vi "Latihan soal UTS 2020.vi"() -> ()   [LabVIEW 2020]
panel:
  out "Warning Counter":i32
  in  "Operator":string
  out "WARNING":bool
  out "Waveform Chart":T1(graph)
  out "START/STOP":bool
  in  "STOP":bool
  in  "START/STOP":bool
  in  "C   or   F":bool
  in  "HIGH Limit":dbl(slide) scale=0.0..100.0
  in  "LOW Limit":dbl(slide) scale=0.0..100.0
  in  "Filename":path
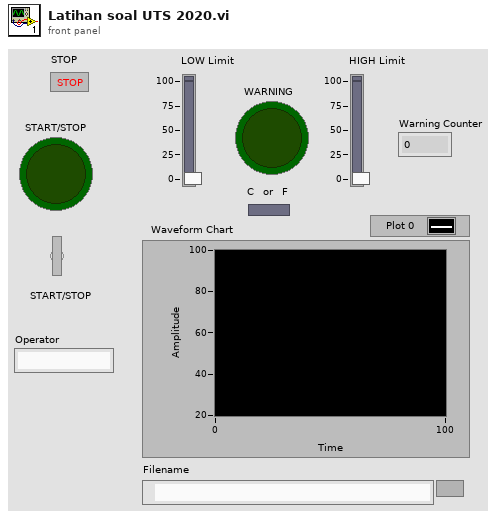
[diagram p1: front panel]
types:
  T1 = cluster{"Temperature (deg F)":dbl, "LOW Limit":dbl, "HIGH Limit":dbl}
  T2 = enum16{"open", "replace", "create", "open or create", "replace or create", "replace or create with confirmation"}
  T3 = cluster{"Y":dbl, "LOW Limit":dbl, "HIGH Limit":dbl}
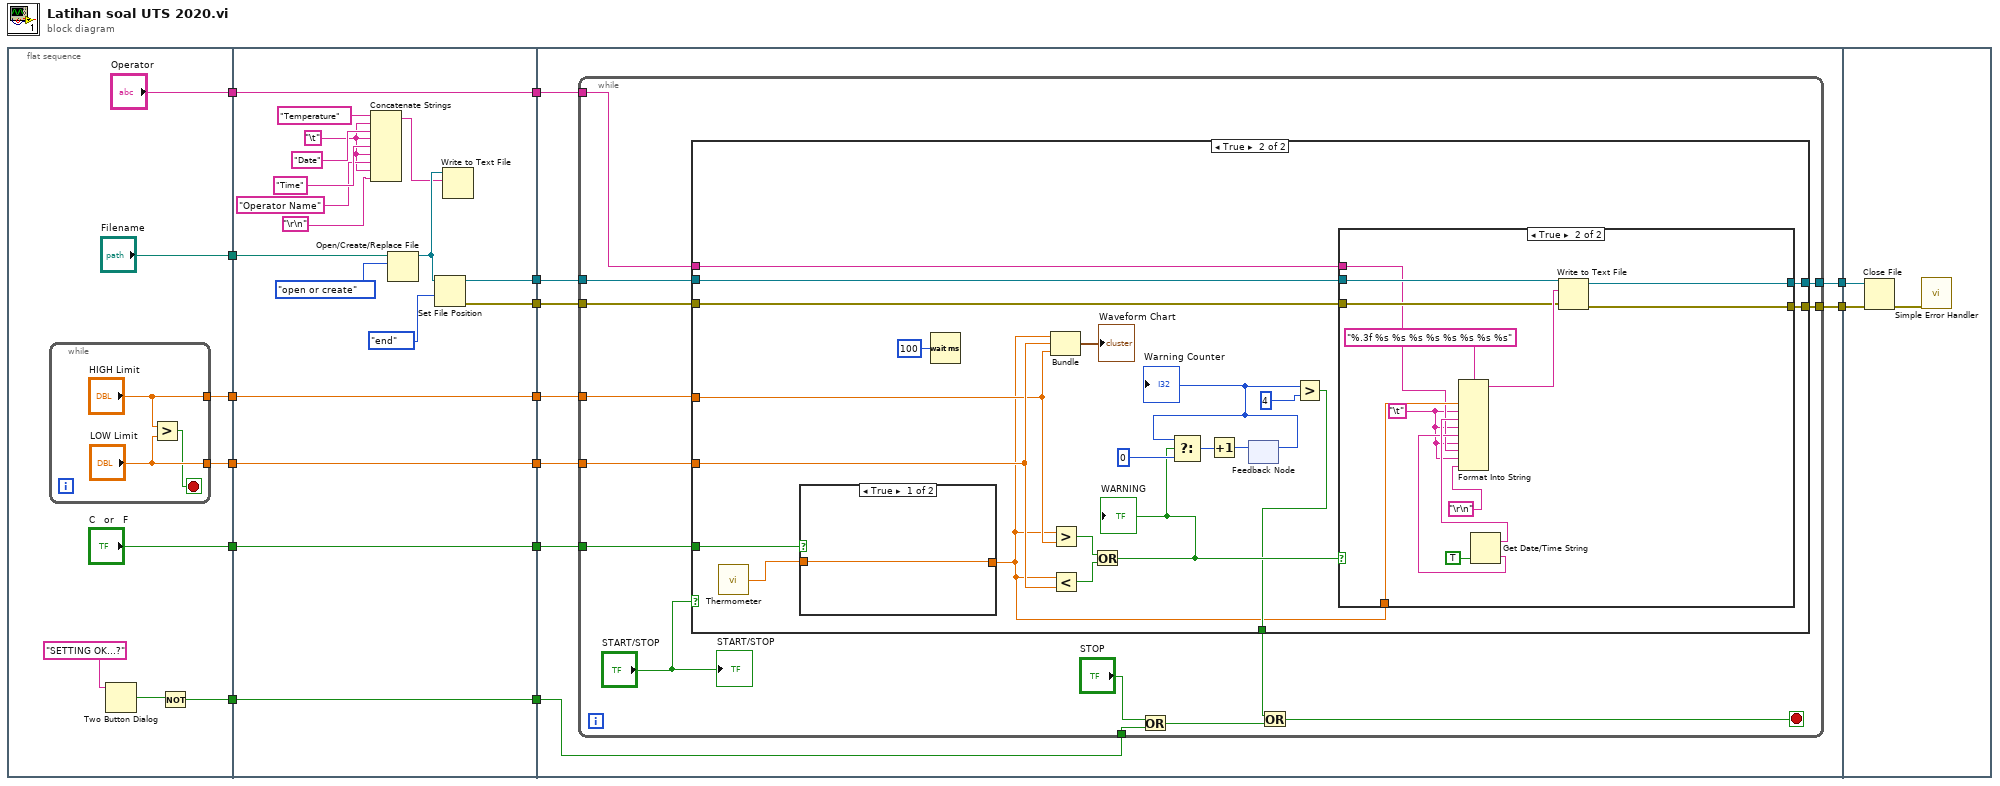
[diagram p0: block diagram]
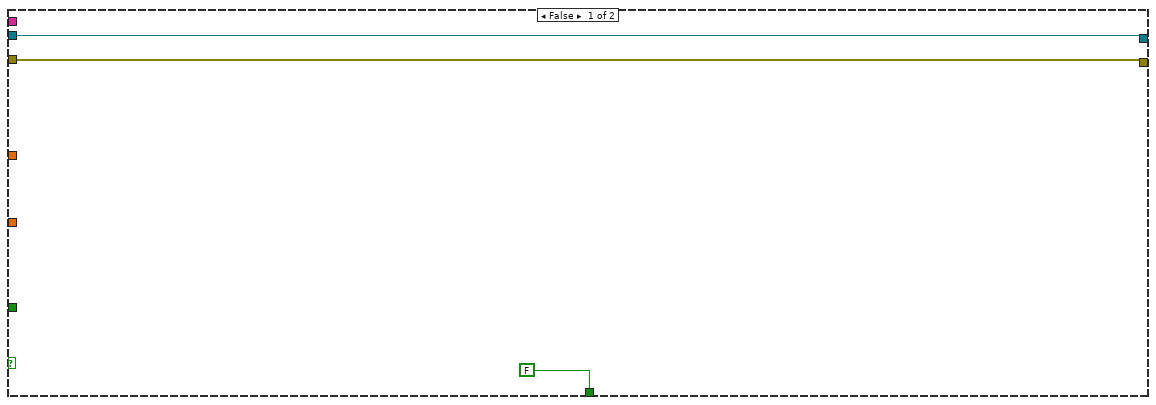
[diagram p2: hidden frame]
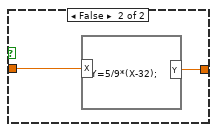
[diagram p4: hidden frame]
diagram:
  n1 = flat-sequence {
    tunnel: ["Filename"] -> w15
    tunnel: ["C   or   F"] -> w13
    tunnel: [w16] -> w11
    tunnel: [w19] -> w9
    tunnel: [w17] -> w3
    tunnel: ["Operator"] -> w1
    tunnel: w15 -> [w44]
    tunnel: [w42] -> w14
    tunnel: w13 -> [w42]
    tunnel: [w28] -> w12
    tunnel: w11 -> [w28]
    tunnel: [w41] -> w10
    tunnel: w9 -> [w41]
    tunnel: [w40] -> w8
    tunnel: [w39] -> w7
    tunnel: [w29] -> w4
    tunnel: w3 -> [w29]
    tunnel: [w36] -> w2
    tunnel: w1 -> [w36]
    tunnel: w14 -> [w53]
    tunnel: w12 -> [w52]
    tunnel: w10 -> [w51]
    tunnel: w8 -> [w50]
    tunnel: w7 -> [w49]
    tunnel: [w48] -> w6
    tunnel: [w47] -> w5
    tunnel: w4 -> [w46]
    tunnel: w2 -> [w45]
    tunnel: w6 -> [w112]
    tunnel: w5 -> [w111]
    frame #0 {
      n2 = while {
        tunnel: ["HIGH Limit"] -> w17
        tunnel: ["LOW Limit"] -> w16
        stop <- w24 stop-if-true
        n3 = Greater?(x="HIGH Limit", y="LOW Limit") -> (0:w24:bool)
      }
      n4 = Two Button Dialog(message="SETTING OK...?") -> (T button?=w20:bool)  [unwired: 2 in]
      n5 = Not(x=w20) -> (.not. x?=w19:bool)
    }
    frame #1 {
      w27 = "\t"
      n6 = Concatenate Strings("Temperature" ("string"), w27, "Date" ("string"), w27, "Time" ("string"), w27, "Operator Name" ("string"), w27, "\r\n") -> (w35:string)
      n7 = Open/Create/Replace File(file path (use dialog)=w44, operation (0:open)=T2."open or create") -> (refnum out=w38:refnum<file>)  [unwired: 4 in, 2 out]
      n8 = Set File Position(refnum=w38, from (0:start)=enum16{"start", "end", "current"}."end") -> (refnum out=w40:refnum<file>, error out=w39:errorcluster)  [unwired: 2 in]
      n9 = Write to Text File(file (use dialog)=w38, text=w35) -> ()  [unwired: 2 in, 3 out]
    }
    frame #2 {
      n10 = while {
        tunnel: w53 -> [w67]
        tunnel: w52 -> [w66]
        tunnel: w51 -> [w64]
        tunnel: w50 -> [w63]
        tunnel: w49 -> [w62]
        tunnel: [w61] -> w48
        tunnel: [w60] -> w47
        tunnel: w46 -> [w59]
        tunnel: w45 -> [w58]
        stop <- w56 stop-if-true
        n11 = case shown="True" "START/STOP" {
          tunnel: w67 -> [_ w91]
          tunnel: w59 -> [_ w76]
          tunnel: w66 -> [_ w81]
          tunnel: w63 -> [w70 w86]
          tunnel: w62 -> [w69 w85]
          tunnel: [w70 w84] -> w61
          tunnel: [w69 w83] -> w60
          tunnel: w58 -> [_ w82]
          tunnel: [FALSE w74] -> w55
          frame False {
          }
          frame True {
            n12 = call "Thermometer.vi"() -> ("Temperature (deg F)"=w71:dbl)  [unwired: 1 in]
            n13 = case shown="True" w91 {
              tunnel: w71 -> [w107 w109]
              tunnel: [w107 w108] -> w72
              frame True {
              }
              frame False {
                n14 = formula code="Y=5/9*(X-32);"("X"=w109) -> ("Y"=w108:dbl)
              }
            }
            n15 = Wait (ms)(milliseconds to wait=u32 100) -> ()  [unwired: 1 out]
            n16 = Bundle("Y"=w72, "LOW Limit"=w81, "HIGH Limit"=w76) -> (→"Waveform Chart":T3)  [unwired: 1 in]
            n17 = Greater?(x=w72, y=w76) -> (0:w90:bool)
            n18 = Less?(x=w72, y=w81) -> (x < y?=w89:bool)
            n19 = Or(x=w90, y=w89) -> (x .or. y?=w75:bool)
            "WARNING" <- w75
            n20 = feedback #1() -> (w73:i32)  [unwired: 1 in]
            "Warning Counter" <- w73
            n21 = Select(t=w73, s=w75, f=0) -> (s? t:f=w79:i32)
            n22 = Increment(x=w79) -> (x+1=w78:i32)
            n23 = feedback-in #1(w78) -> ()
            n24 = Greater?(x=w73, y=4) -> (0:w74:bool)
            n25 = case shown="True" w75 {
              tunnel: w72 -> [_ w105]
              tunnel: w86 -> [w92 w103]
              tunnel: w85 -> [w93 w102]
              tunnel: [w92 w101] -> w84
              tunnel: [w93 w100] -> w83
              tunnel: w82 -> [_ w95]
              frame False {
              }
              frame True {
                w94 = "\t"
                n26 = Get Date/Time String(want seconds? (F)=TRUE) -> (date string=w98:string, time string=w97:string)  [unwired: 2 in]
                n27 = Format Into String "Format Into String"(format string="%.3f %s %s %s %s %s %s %s %s", w105, w94, w98, w94, w97, w94, w95, w94, "\r\n") -> (resulting string=w104:string)  [unwired: 2 in, 1 out]
                n28 = Write to Text File(file (use dialog)=w103, text=w104, error in=w102) -> (refnum out=w101:refnum<file>, error out=w100:errorcluster)  [unwired: 1 in, 1 out]
              }
            }
          }
        }
        n29 = Or(x="STOP", y=w64) -> (x .or. y?=w57:bool)
        n30 = Or(x=w55, y=w57) -> (x .or. y?=w56:bool)
        "START/STOP" <- "START/STOP"
      }
    }
    frame #3 {
      n31 = Close File(refnum=w112, error in=w111) -> (error out=w110:errorcluster)  [unwired: 1 out]
      n32 = call <vilib>:"Simple Error Handler.vi"("error in (no error)"=w110) -> ()  [unwired: 4 in, 5 out]
    }
  }
